vi "Measure_G.vi"(6 "Internal":bool, 7 "All":bool, 8 "error in (no error)":errorcluster, 9 "WCM_correction":bool, 10 "# scans":i32=-1, 11 "Control-Client in":refnum<class "Control-Client.lvclass">) -> (0 "error out":errorcluster, 3 "Control-Client out":refnum<class "Control-Client.lvclass">)   [LabVIEW 2018, in "Control-Client.lvclass"]
uses:
  Control-Client.lvclass
  dependecies/ControlsVIs/Clusters-def/Message types.ctl
  dependecies/ControlsVIs/Clusters-def/SERVER-Commands.ctl
  dependecies/ControlsVIs/Clusters-def/Det-Read.ctl
  dependecies/ControlsVIs/Clusters-def/Parameters_measurement_def.ctl
  Control-Client.lvclass/Control-Client.ctl
  Control-Server/Control-Server.lvclass
  Detector/Detector.lvclass
  Experiments/Experiment.lvclass
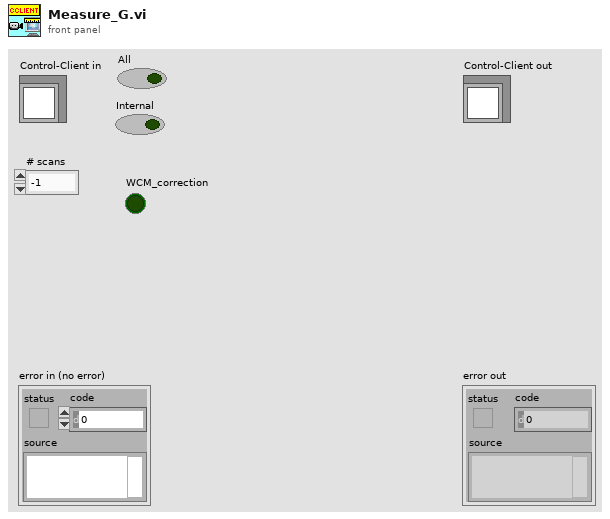
[diagram p1: front panel]
types:
  T1 = typedef "Detector.lvclass/Det-Read.ctl" = cluster{"# scans":i32, "All":bool, "Parameters of measurement":T2}
  T2 = typedef "Parameters_measurement_def.ctl" = cluster{"ODmin":dbl, "ODmax":dbl, "Aq contol":enum32{"fixed", "automatic", "fixed-auto"}, "Wavelength_fix_index":i32, "WCM_limits":cluster{"WCM_min":dbl, "WCM_max":dbl, "WCM_value":dbl}, "WCM_corrections":bool, "#cycles max":i32}
  T3 = typedef "Control-Server.lvclass/SERVER-Commands.ctl" = string
  T4 = typedef "Message types.ctl" = string
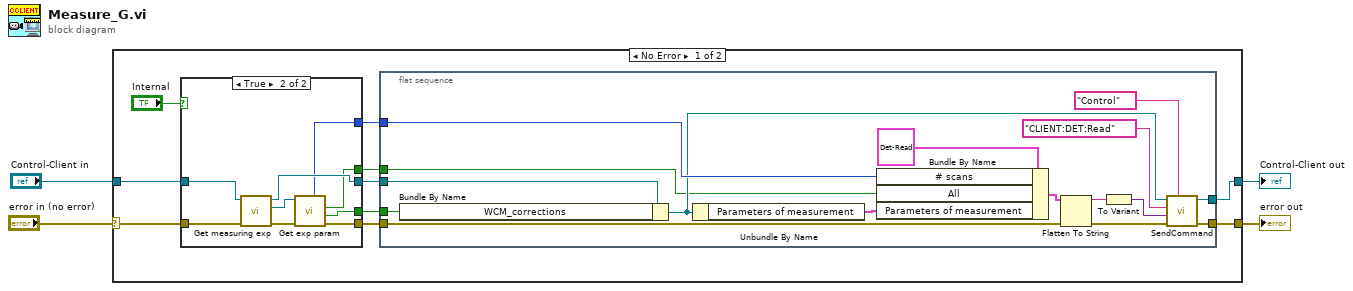
[diagram p0: block diagram]
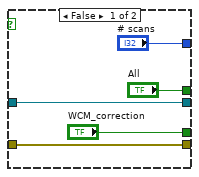
[diagram p2: hidden frame]
diagram:
  n1 = case shown="No Error" "error in (no error)" {
    selector: "error in (no error)" -> [w13 w46]
    tunnel: [w10 w46] -> w3
    tunnel: [w9 w45] -> w1
    tunnel: "Control-Client in" -> [w12 w45]
    frame No Error {
      n2 = case shown="True" "Internal" {
        tunnel: ["# scans" w40] -> w14
        tunnel: w13 -> [w35 w38]
        tunnel: w12 -> [w34 w44]
        tunnel: [w35 w39] -> w11
        tunnel: [w34 w41] -> w8
        tunnel: ["All" w37] -> w6
        tunnel: ["WCM_correction" w36] -> w5
        frame False {
        }
        frame True {
          n3 = call "Get measuring exp.vi"("error in (no error)"=w38, "Control-Client in"=w44) -> ("error out"=w43:errorcluster, "Measured experiment"=w42:refnum<class "Experiment.lvclass">, "Control-Client out"=w41:refnum<class "Control-Client.lvclass">)  [unwired: 7 in]
          n4 = call "Get exp param.vi"("error in (no error)"=w43, "Experiment in"=w42) -> ("error out"=w39:errorcluster, "WCM_correction"=w36:bool, "All"=w37:bool, "#pp"=w40:i32)  [unwired: 5 in, 1 out]
        }
      }
      n5 = flat-sequence {
        tunnel: w14 -> [w27]
        tunnel: w11 -> [w26]
        tunnel: [w20] -> w10
        tunnel: [w21] -> w9
        tunnel: w8 -> [w18]
        tunnel: w6 -> [w16]
        tunnel: w5 -> [w15]
        frame #0 {
          n6 = Bundle By Name(cluster=w18, "WCM_corrections"=w15) -> (w17:refnum<class "Control-Client.lvclass">)
          n7 = Unbundle By Name(w17) -> ("Parameters of measurement"=w19:T2)
          n8 = Bundle By Name(cluster=T1 {"# scans"=0, "All"=FALSE, "Parameters of measurement"={"ODmin"=0.0, "ODmax"=0.0, "Aq contol"=enum."fixed", "Wavelength_fix_index"=640, "WCM_limits"={"WCM_min"=0.0, "WCM_max"=0.0, "WCM_value"=0.0}, "WCM_corrections"=FALSE, "#cycles max"=5}}, "# scans"=w27, "All"=w16, "Parameters of measurement"=w19) -> (w25:T1)
          n9 = Flatten To String(anything=w25, error in (no error)=w26) -> (data string=w24:string, error out=w23:errorcluster)  [unwired: 2 in, 1 out]
          n10 = To Variant(anything=w24) -> (Variant=w28:variant)
          n11 = call "SendCommand.vi"("Message type"=T4 "Control", "error in (no error)"=w23, "data"=w28, "Command"=T3 "CLIENT:DET:Read" ("Commands"), "Control-Client in"=w17) -> ("error out"=w20:errorcluster, "Control-Client out"=w21:refnum<class "Control-Client.lvclass">)  [unwired: 5 in]
        }
      }
    }
    frame Error {
    }
  }
  "error out" <- w3
  "Control-Client out" <- w1
